vi "Streamed Data Viewer.vi"() -> ()   [LabVIEW 2013]
doc: "Use this template to build a user interface event handler design pattern. Use this pattern for dialog boxes and other user interfaces. You also can create and execute user-defined events that the VI can handle the same way as user interface events."
uses:
  <vilib>/Waveform/WDTFileIO.llb/ Write Waveforms to File (1D).vi
  <vilib>/Waveform/WDTFileIO.llb/Export Waveforms To Spreadsheet File (1D).vi
  <vilib>/Waveform/WDTOps.llb/WDT Append Waveforms DBL.vi
panel:
  in  "Save CSV Reduced":bool
  in  "Save CSV":bool
  out "Delta Y\nReduced Waveform Data":dbl format="%#.6g"
  out "Delta X\nReduced Waveform Data":dbl format="%#.6g"
  out "Delta Y\nWaveform Data":dbl format="%#.6g"
  out "Delta X\nWaveform Data":dbl format="%#.6g"
  out "offset (in bytes)":i64
  in  "Input Has Array Size":bool
  in  "Subtract":bool
  in  "Convert":bool
  out "Records\nLoaded":u32
  in  "# Channels":u32=7
  in  "End Record":u32
  in  "Start Record":u32
  in  "Save Reduced DBL":bool
  in  "Save DBL":bool
  in  "Save WFM Reduced":bool
  in  "Save WFM":bool
  in  "Reduced Data Out Directory":path
  in  "Data Out Directory":path
  in  "Reduced Records":waveform(dbl)[][](array[waveform])
  out "Reduced Waveform Data":waveform(dbl)[](graph)
  out "RF Pulse Indicies":u32[][](array[numeric])
  in  "Displayed Record":u32(slide)=1 min=1 step=1 scale=1.0..27.0
  in  "Records":waveform(dbl)[][](array[waveform])
  out "Waveform Data":waveform(dbl)[](graph)
  out "Record Count":u32
  in  "Sampling Rate":u32=500000
  in  "Record Channel Size":bool=TRUE
  in  "Path":path
  in  "Load":bool
  in  "stop":bool
  # "51200"
  # "51200 x 3"
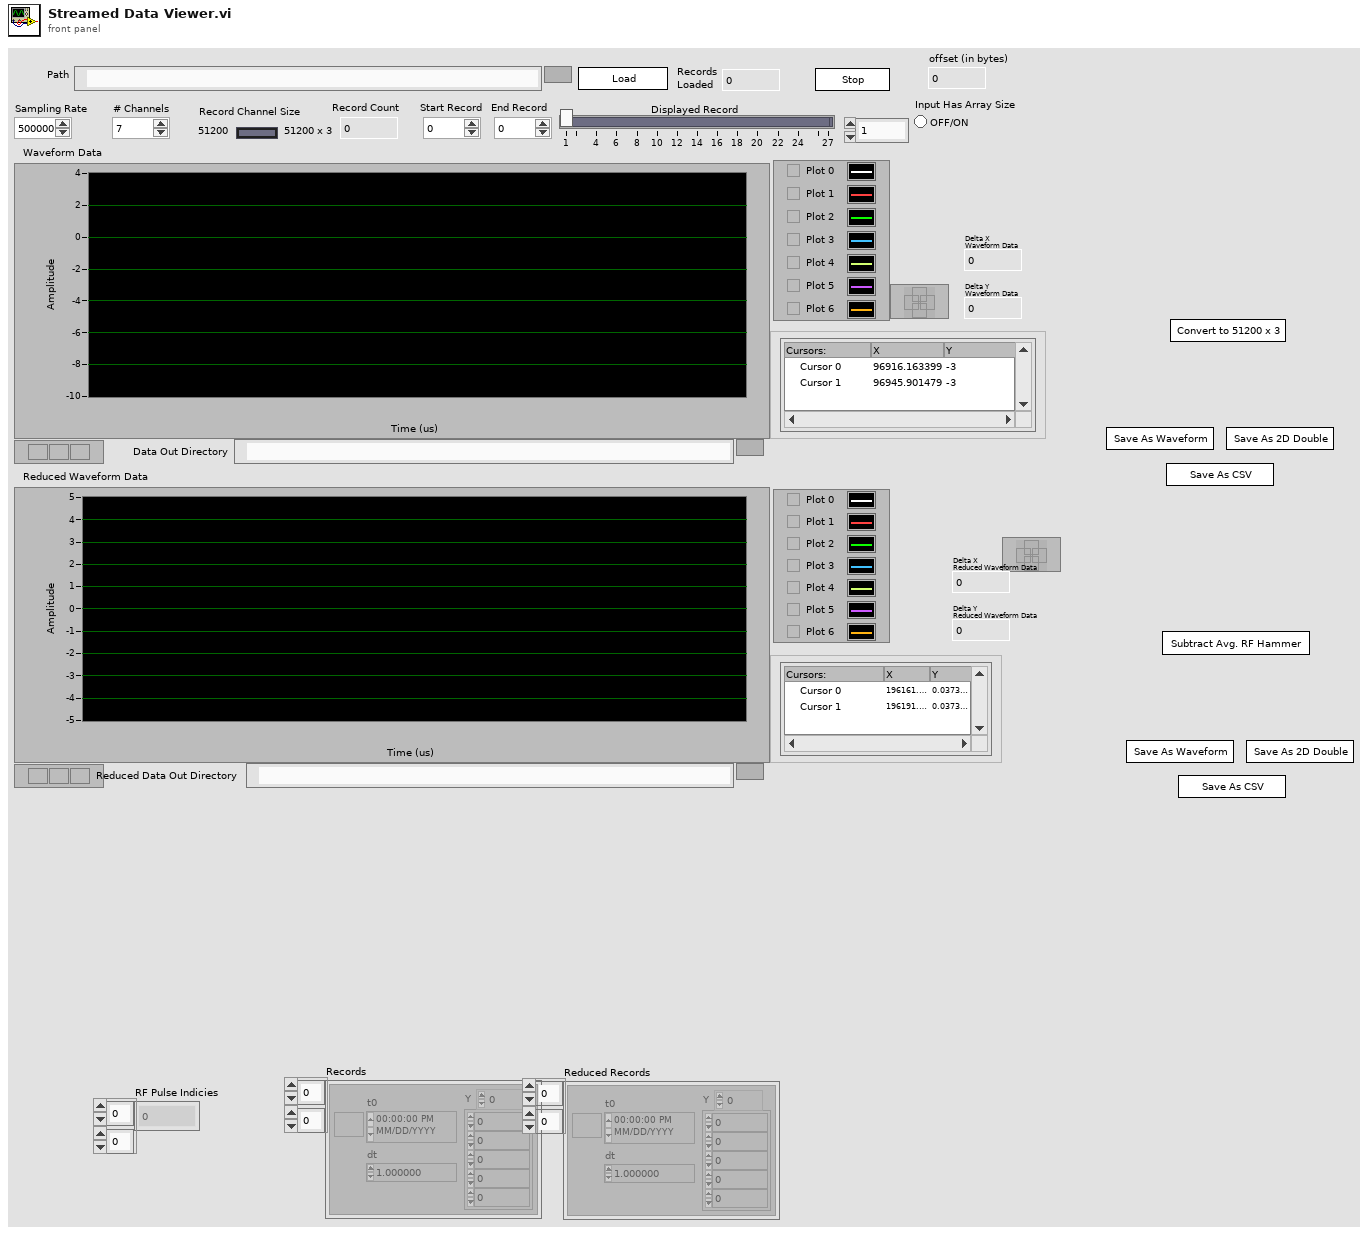
[diagram p1: front panel]
types:
  T1 = enum16{"big-endian, network order", "native, host order", "little-endian"}
  T2 = enum16{"open", "replace", "create", "open or create", "replace or create", "replace or create with confirmation"}
  T3 = typedef "LVCursorListTypeDef.ctl" = cluster{"Name":string, "Color":u32, "Style":u8, "Point Style":u8, "Name Visible":bool, "Allow Drag":bool, "Cursor Mode":u32, "Plot":i32, "Index":i32, "Position":cluster{"X":dbl, "Y":dbl}, "X Scale":u32, "Y Scale":u32, "Watch Plots":i32[], "Watch All Plots":bool, "Plot Area":i32, "Label Offset":cluster{"X":dbl, "Y":dbl}}[]
  T4 = cluster{"Name":string, "Color":u32, "Style":u8, "Point Style":u8, "Name Visible":bool, "Allow Drag":bool, "Cursor Mode":u32, "Plot":i32, "Index":i32, "Position":cluster{"X":dbl, "Y":dbl}, "X Scale":u32, "Y Scale":u32, "Watch Plots":i32[], "Watch All Plots":bool, "Plot Area":i32, "Label Offset":cluster{"X":dbl, "Y":dbl}}
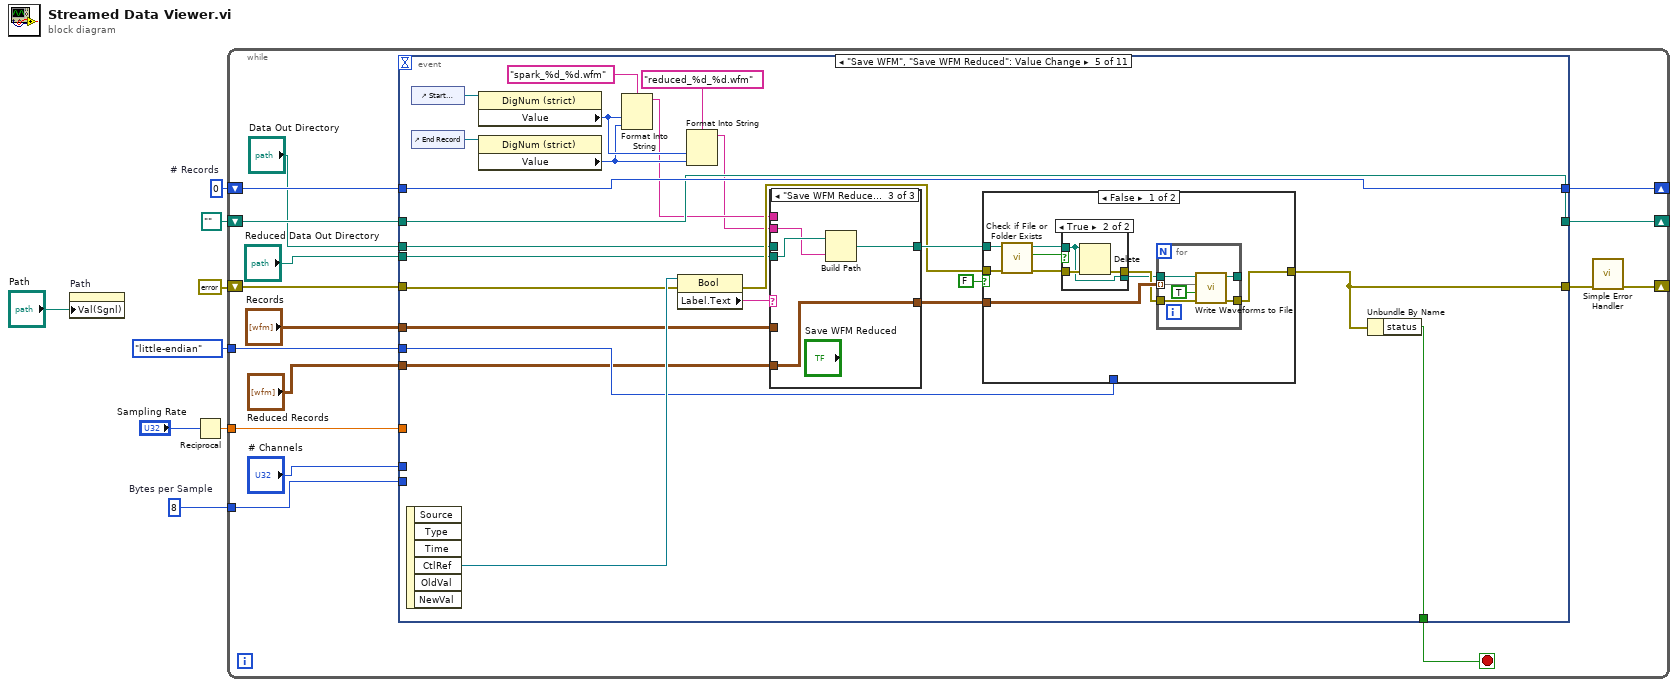
[diagram p0: block diagram]
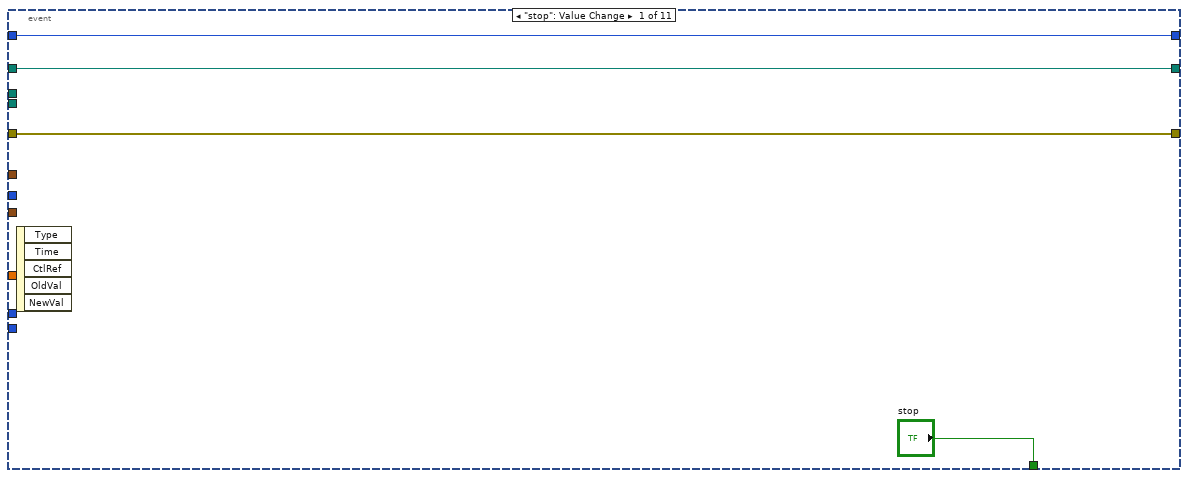
[diagram p2: hidden frame]
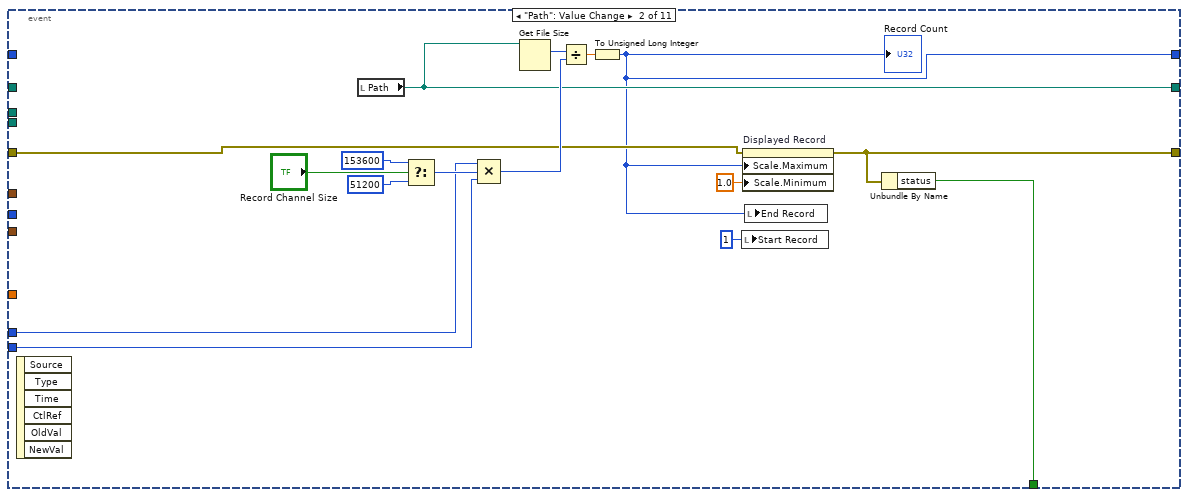
[diagram p3: hidden frame]
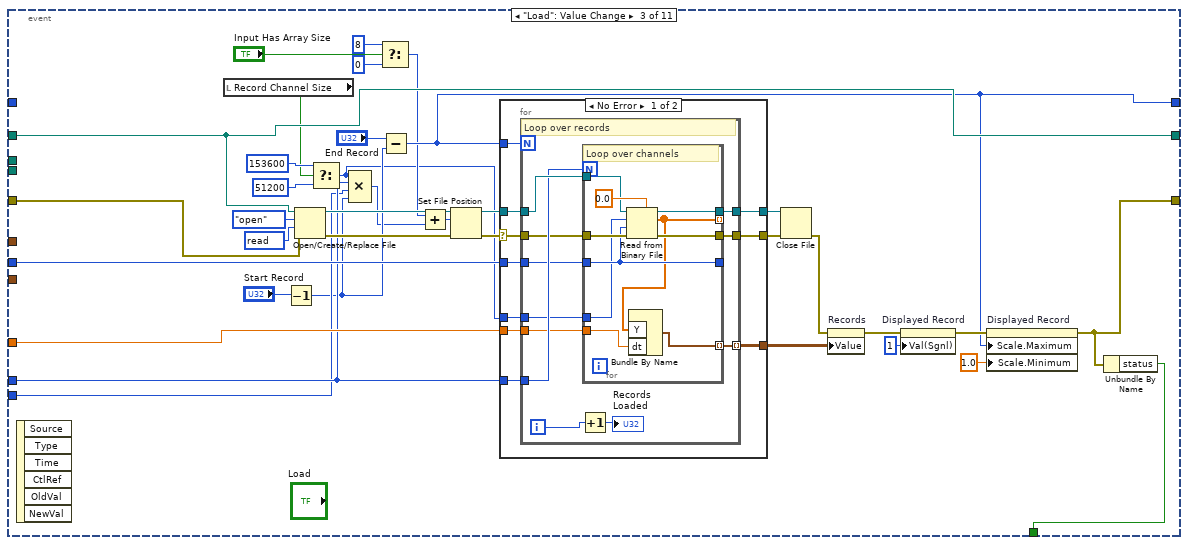
[diagram p4: hidden frame]
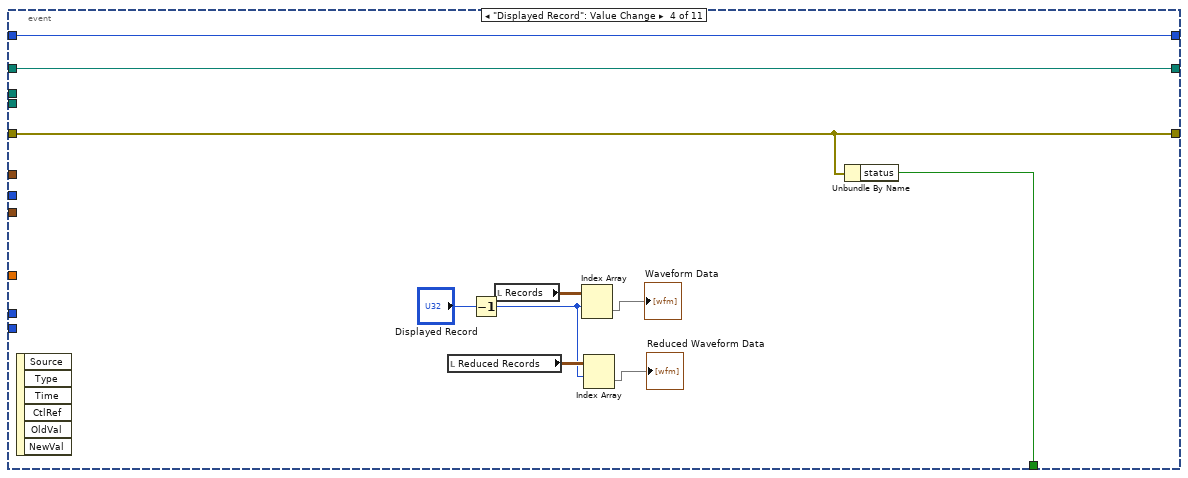
[diagram p6: hidden frame]
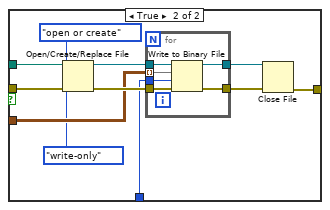
[diagram p8: hidden frame]
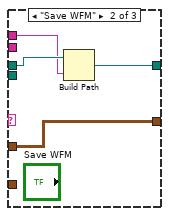
[diagram p10: hidden frame]
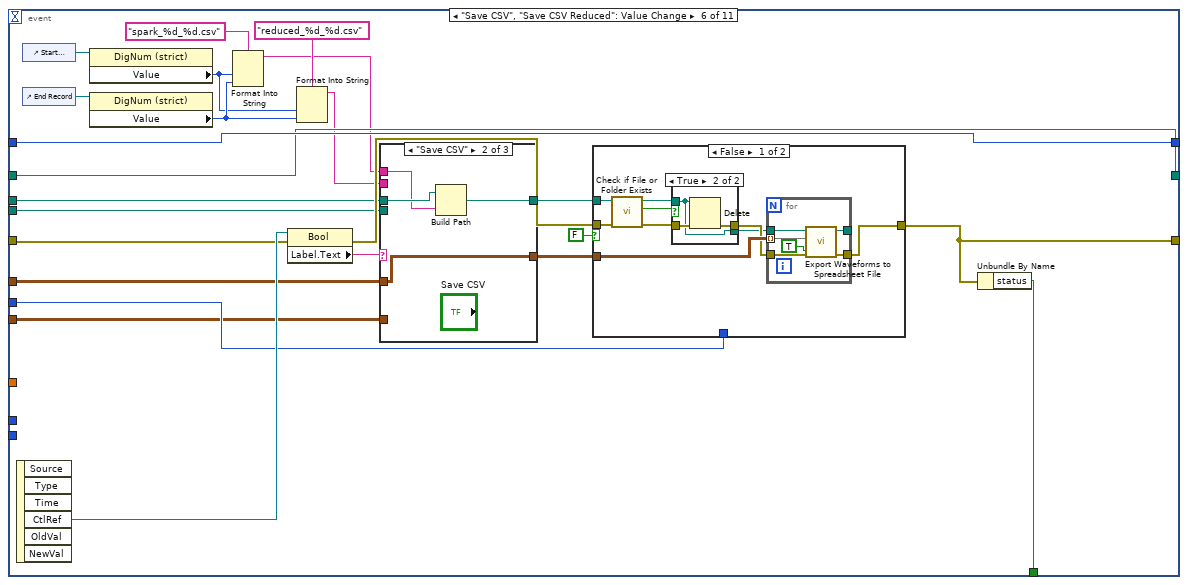
[diagram p11: hidden frame]
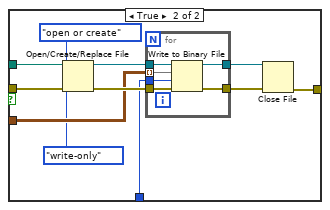
[diagram p13: hidden frame]
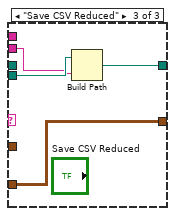
[diagram p15: hidden frame]
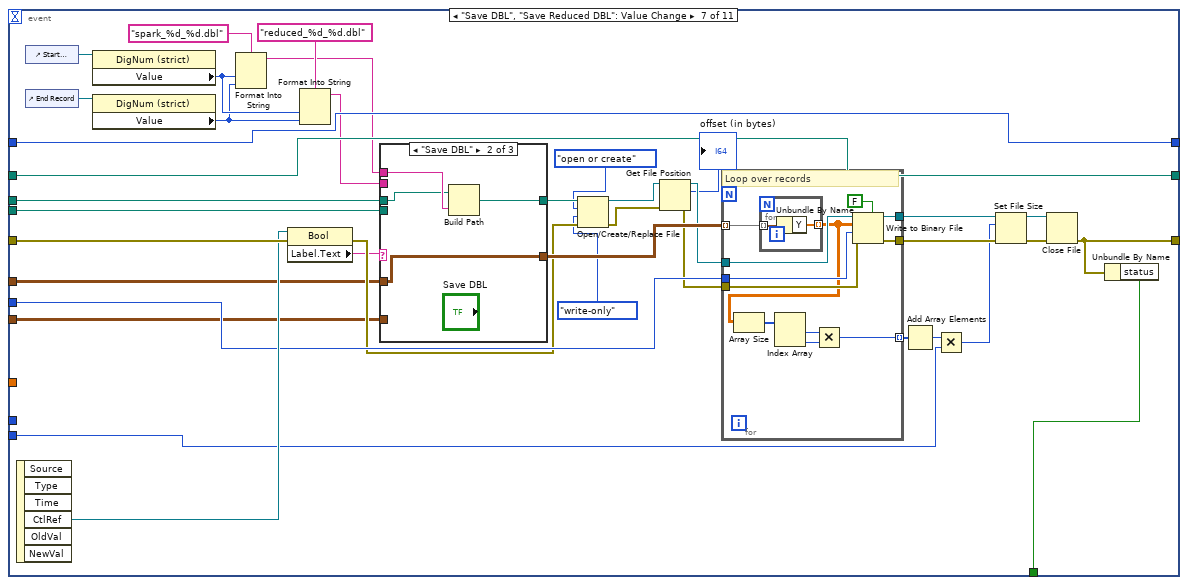
[diagram p16: hidden frame]
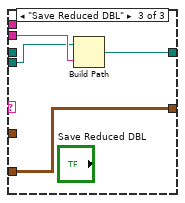
[diagram p18: hidden frame]
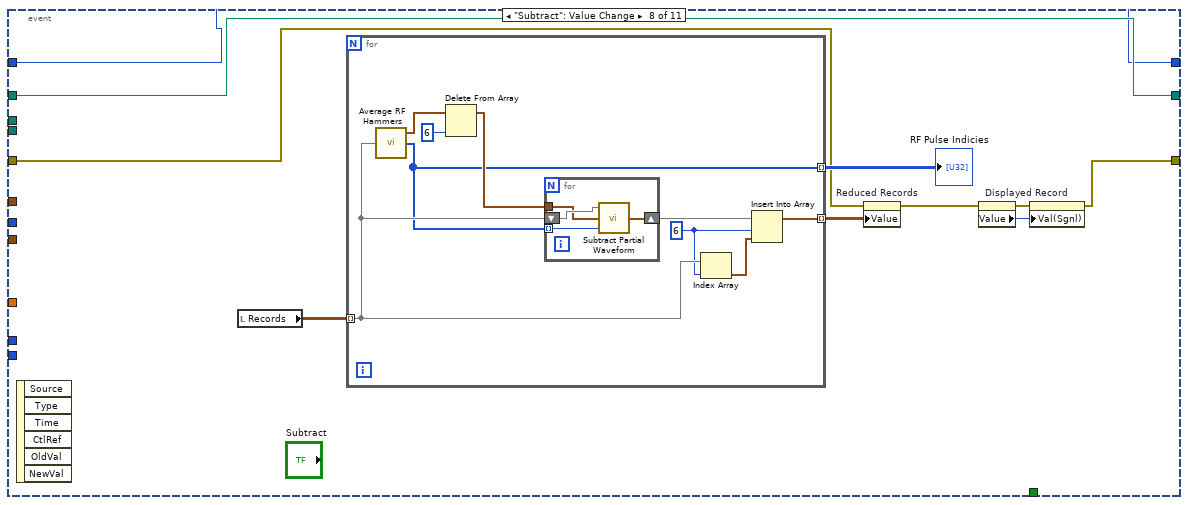
[diagram p19: hidden frame]
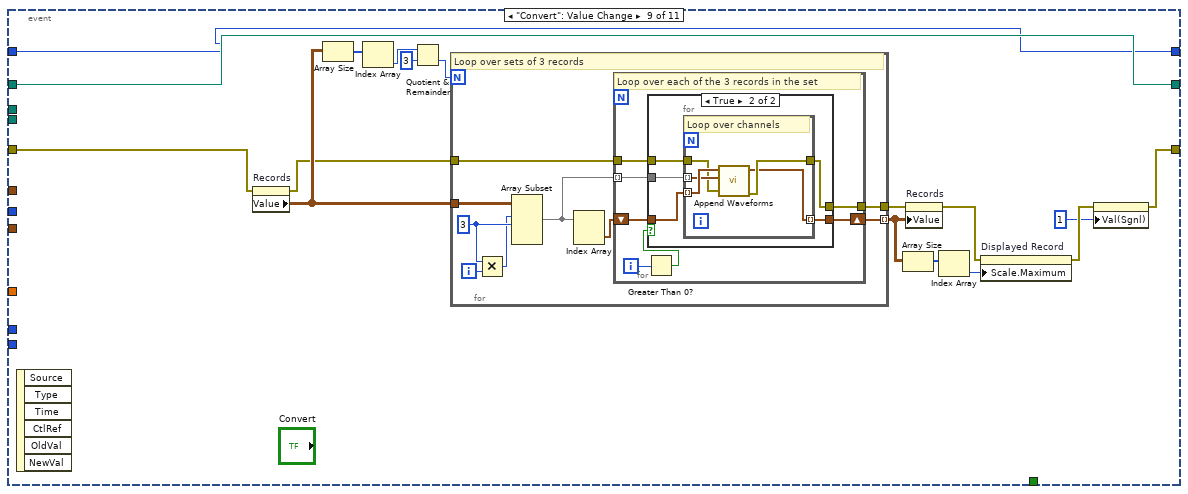
[diagram p20: hidden frame]
diagram:
  w6 = u32 8  # Bytes per Sample
  w8 = u32 0  # # Records
  n1 = property on="Path" class="Path"("Val(Sgnl)"="Path") -> ()  [unwired: 2 in, 2 out]
  n2 = Reciprocal(x="Sampling Rate") -> (1/x=w4:dbl)
  n3 = while {
    shift-right: [w23] -> _
    shift-left: w8 -> [w22]
    shift-right: [w21] -> _
    shift-left: path "" ("Path") -> [w20]
    tunnel: w6 -> [w19]
    tunnel: w4 -> [w18]
    tunnel: T1."little-endian" ("byte order (0:big-endian, network order)") -> [w17]
    shift-right: [w13] -> _
    shift-left: errorcluster {"status"=FALSE, "code"=0, "source"=""} ("error out") -> [w16]
    stop <- w24 stop-if-true
    n4 = event shown="[4] \"Save WFM\", \"Save WFM Reduced\": Value Change" {
      selector: _ -> [_ _ _ _ _ _ _ _ _ _ _]
      dyn-events: _ -> [_ _ _ _ _ _ _ _ _ _ _]
      timeout: _ -> [_ _ _ _ _ _ _ _ _ _ _]
      tunnel: ["stop" w31 w75 w114 w137 w206 w289 _ _ _ _] -> w24
      tunnel: [w26 w29 w55 w119 w141 w210 w294 w322 w353 w393 w409] -> w23
      tunnel: w22 -> [w26 _ _ w119 w141 w210 w294 w322 w353 w393 w409]
      tunnel: [w27 w37 w77 w120 w140 w209 w293 w323 w354 w392 w408] -> w21
      tunnel: w20 -> [w27 _ w77 w120 w140 w209 w293 w323 w354 w392 w408]
      tunnel: "# Channels" -> [_ w39 w64 _ _ _ _ _ _ _ _]
      tunnel: w19 -> [_ w38 w63 _ _ _ w275 _ _ _ _]
      tunnel: w18 -> [_ _ w79 _ _ _ _ _ _ _ _]
      tunnel: w17 -> [_ _ w78 _ w139 w208 w295 _ _ _ _]
      tunnel: [w25 w32 w60 w115 w138 w207 w290 w324 w355 w390 w406] -> w14
      tunnel: w16 -> [w25 w34 w71 w115 w146 w215 w299 w326 w356 w391 w407]
      tunnel: "Data Out Directory" -> [_ _ _ _ w135 w204 w273 _ _ _ _]
      tunnel: "Reduced Data Out Directory" -> [_ _ _ _ w134 w203 w272 _ _ _ _]
      tunnel: "Records" -> [_ _ _ _ w133 w202 w271 _ _ _ _]
      tunnel: "Reduced Records" -> [_ _ _ _ w132 w201 w270 _ _ _ _]
      event "stop": Value Change {
        n5 = event-data() -> ()  [unwired: 1 in, 5 out]
      }
      event "Path": Value Change {
        n6 = event-data() -> ()  [unwired: 1 in, 6 out]
        n7 = local read "Path"() -> (w37:path)
        n8 = Select(t=u32 153600, s="Record Channel Size", f=u32 51200) -> (s? t:f=w40:u32)
        n9 = Compound Arithmetic op=MULTIPLY(w39, w40, w38) -> (w41:u32)
        n10 = Get File Size(file=w37) -> (size (in bytes)=w42:i64)  [unwired: 1 in, 2 out]
        n11 = Divide(x=w42, y=w41) -> (x/y=w43:dbl)
        n12 = To Unsigned Long Integer(number=w43) -> (unsigned 32bit integer=w29:u32)
        "Record Count" <- w29
        n13 = local write "Start Record"(u32 1 ("Start Record")) -> ()
        n14 = property on="Displayed Record" class="Slide (strict)"(error in=w34, "Scale.Maximum"=w29, "Scale.Minimum"=1.0 ("Scale.Range:Minimum")) -> (error out=w32:errorcluster)  [unwired: 1 in, 1 out]
        n15 = local write "End Record"(w29) -> ()
        n16 = Unbundle By Name(w32) -> ("status"=w31:bool)
      }
      event "Load": Value Change {
        w80 = u32 2147483648 items=["read"=2147483648, "write"=1073741824, "read & write"=3221225472, "execute"=536870912, "all"=268435456] ("desired access (read & write)")
        n17 = event-data() -> ()  [unwired: 1 in, 6 out]
        n18 = local read "Record Channel Size"() -> (w65:bool)
        n19 = Decrement(x="Start Record") -> (x-1=w56:u32)
        n20 = Open/Create/Replace File(file path (use dialog)=w77, error in=w71, operation (0:open)=T2."open", access (0:read/write)=w80) -> (refnum out=w69:refnum<file>, error out=w70:errorcluster)  [unwired: 2 in, 1 out]
        n21 = Select(t=u32 153600, s=w65, f=u32 51200) -> (s? t:f=w48:u32)
        n22 = Compound Arithmetic op=MULTIPLY(w48, w64, w63, w56) -> (w50:u32)
        n23 = Select(t=u32 8, s="Input Has Array Size", f=u32 0) -> (s? t:f=w49:u32)
        n24 = Subtract(x="End Record", y=w56) -> (x-y=w55:u32)
        n25 = Add(x=w49, y=w50) -> (x+y=w51:u32)
        n26 = Set File Position(offset (in bytes) (0)=w51, refnum=w69, error in=w70) -> (refnum out=w68:refnum<file>, error out=w59:errorcluster)  [unwired: 1 in]
        n27 = case shown="No Error" w59 {
          selector: w59 -> [w81 w112]
          tunnel: w48 -> [w90 _]
          tunnel: w79 -> [w89 _]
          tunnel: w78 -> [w88 _]
          tunnel: [w87 w113] -> w47
          tunnel: [w86 _] -> w74
          tunnel: [w85 w112] -> w46
          tunnel: w68 -> [w84 w113]
          tunnel: w64 -> [w83 _]
          tunnel: w55 -> [w82 _]
          frame No Error {
            n28 = for {
              N: w82 -> [_]
              tunnel: w84 -> [w101]
              tunnel: w83 -> [w100]
              tunnel: w90 -> [w99]
              tunnel: w81 -> [w98]
              tunnel: w89 -> [w97]
              tunnel: w88 -> [w96]
              tunnel: [w95] -> w87
              tunnel: [w94] -> w85
              tunnel: [w93] -> w86 mode=indexing
              i -> [w91]
              # "Loop over records"
              n29 = Increment(x=w91) -> (x+1=→"Records\nLoaded":i32)
              n30 = for {
                N: w100 -> [_]
                tunnel: [w111] -> w93 mode=indexing
                tunnel: w101 -> [w109]
                tunnel: w99 -> [w103]
                tunnel: w98 -> [w108]
                tunnel: w97 -> [w107]
                tunnel: w96 -> [w105]
                tunnel: [w106] -> w94
                tunnel: [w105] -> _
                tunnel: [w104] -> w95
                tunnel: [w102] -> _ mode=indexing
                # "Loop over channels"
                n31 = Read from Binary File(5:0.0, 8:w108, 9:w105, 10:w103, 11:w109) -> (0:w106:errorcluster, 2:w102:dbl[], 3:w104:refnum<file>)  [unwired: 1 in, 1 out]
                n32 = Bundle By Name("Y"=w102, "dt"=w107) -> (w111:waveform(dbl))  [unwired: 1 in]
              }
            }
          }
          frame Error {
          }
        }
        n33 = Close File(refnum=w47, error in=w46) -> (error out=w45:errorcluster)  [unwired: 1 out]
        n34 = property on="Records" class="Arr (strict)"(error in=w45, "Value"=w74) -> (error out=w72:errorcluster)  [unwired: 1 in, 1 out]
        n35 = property on="Displayed Record" class="Slide (strict)"(error in=w72, "Val(Sgnl)"=u32 1 ("Value (Signaling)")) -> (error out=w61:errorcluster)  [unwired: 1 in, 1 out]
        n36 = property on="Displayed Record" class="Slide (strict)"(error in=w61, "Scale.Maximum"=w55, "Scale.Minimum"=1.0 ("Scale.Range:Minimum")) -> (error out=w60:errorcluster)  [unwired: 1 in, 1 out]
        n37 = Unbundle By Name(w60) -> ("status"=w75:bool)
      }
      event "Displayed Record": Value Change {
        n38 = event-data() -> ()  [unwired: 1 in, 6 out]
        n39 = local read "Reduced Records"() -> (w118:waveform(dbl)[][])
        n40 = Decrement(x="Displayed Record") -> (x-1=w117:u32)
        n41 = local read "Records"() -> (w123:waveform(dbl)[][])
        n42 = Index Array(array=w123, index (row)=w117) -> (element=→"Waveform Data":waveform(dbl)[])  [unwired: 1 in]
        n43 = Index Array(array=w118, index (row)=w117) -> (element=→"Reduced Waveform Data":waveform(dbl)[])  [unwired: 1 in]
        n44 = Unbundle By Name(w115) -> ("status"=w114:bool)
      }
      event "Save WFM", "Save WFM Reduced": Value Change {
        n45 = event-data() -> ("CtlRef"=w147:refnum<vi>)  [unwired: 1 in, 5 out]
        n46 = control-ref of="Start Record"() -> (w131:refnum<vi>)
        n47 = control-ref of="End Record"() -> (w130:refnum<vi>)
        n48 = property class="DigNum (strict)"(reference=w131) -> ("Value"=w127:u32)  [unwired: 1 in, 2 out]
        n49 = property class="DigNum (strict)"(reference=w130) -> ("Value"=w126:u32)  [unwired: 1 in, 2 out]
        n50 = Format Into String(format string="spark_%d_%d.wfm", w127, w126) -> (resulting string=w125:string)  [unwired: 2 in, 1 out]
        n51 = property class="Bool"(reference=w147, error in=w146) -> (error out=w143:errorcluster, "Label.Text"=w145:string)  [unwired: 1 out]
        n52 = Format Into String(format string="reduced_%d_%d.wfm", w127, w126) -> (resulting string=w124:string)  [unwired: 2 in, 1 out]
        n53 = case shown="\"Save WFM Reduced\"" w145 {
          tunnel: [_ w185 w189] -> w144
          tunnel: [_ w188 w192] -> w142
          tunnel: w135 -> [_ w187 _]
          tunnel: w134 -> [_ _ w191]
          tunnel: w133 -> [_ w188 _]
          tunnel: w132 -> [_ _ w192]
          tunnel: w125 -> [_ w186 _]
          tunnel: w124 -> [_ _ w190]
          frame Default {
            # "NO-OP"
          }
          frame "Save WFM" {
            n54 = Build Path(base path=w187, name or relative path=w186) -> (appended path=w185:path)
          }
          frame "Save WFM Reduced" {
            n55 = Build Path(base path=w191, name or relative path=w190) -> (appended path=w189:path)
          }
        }
        n56 = case shown="False" FALSE {
          tunnel: w144 -> [w151 w178]
          tunnel: w143 -> [w152 w177]
          tunnel: w142 -> [w156 w175]
          tunnel: w139 -> [_ w171]
          tunnel: [w154 w170] -> w138
          frame False {
            n57 = call <vilib>:"Check if File or Folder Exists.vi"("error in (no error)"=w152, "path"=w151) -> ("error out"=w149:errorcluster, "file or folder exists?"=w148:bool, "dup path"=w150:path)  [unwired: 7 in]
            n58 = case shown="True" w148 {
              tunnel: w150 -> [w157 w159]
              tunnel: w149 -> [w158 w161]
              tunnel: [w157 w159] -> w153
              tunnel: [w158 w160] -> w155
              frame False {
              }
              frame True {
                n59 = Delete(path (use dialog)=w159, error in=w161) -> (error out=w160:errorcluster)  [unwired: 3 in, 2 out]
              }
            }
            n60 = for {
              tunnel: w155 -> [w167]
              tunnel: w156 -> [w163] mode=indexing
              tunnel: [w166] -> w154
              tunnel: [w165] -> _
              tunnel: w153 -> [w164]
              n61 = call-poly <vilib>:"Write Waveforms to File.vi"("error in (no error)"=w167, "append to file? (new file:F)"=TRUE, "waveform array"=w163, "file path (dialog if empty)"=w164) -> ("error out"=w166:errorcluster, "new file path (Not A Path if cancelled)"=w165:path)  [unwired: 6 in]
            }
          }
          frame True {
            n62 = Open/Create/Replace File(file path (use dialog)=w178, error in=w177, operation (0:open)=T2."open or create", access (0:read/write)=enum16{"read/write", "read-only", "write-only"}."write-only") -> (refnum out=w172:refnum<file>, error out=w176:errorcluster)  [unwired: 2 in, 1 out]
            n63 = for {
              tunnel: w176 -> [w184]
              tunnel: w175 -> [w183] mode=indexing
              tunnel: [w182] -> w174
              tunnel: [w181] -> w173
              tunnel: w172 -> [w180]
              tunnel: w171 -> [w179]
              n64 = Write to Binary File(file (use dialog)=w180, data=w183, error in=w184, 9:w179) -> (refnum out=w181:refnum<file>, error out=w182:errorcluster)  [unwired: 2 in, 1 out]
            }
            n65 = Close File(refnum=w173, error in=w174) -> (error out=w170:errorcluster)  [unwired: 1 out]
          }
        }
        n66 = Unbundle By Name(w138) -> ("status"=w137:bool)
      }
      event "Save CSV", "Save CSV Reduced": Value Change {
        n67 = event-data() -> ("CtlRef"=w216:refnum<vi>)  [unwired: 1 in, 5 out]
        n68 = control-ref of="Start Record"() -> (w196:refnum<vi>)
        n69 = control-ref of="End Record"() -> (w197:refnum<vi>)
        n70 = property class="DigNum (strict)"(reference=w196) -> ("Value"=w199:u32)  [unwired: 1 in, 2 out]
        n71 = property class="DigNum (strict)"(reference=w197) -> ("Value"=w200:u32)  [unwired: 1 in, 2 out]
        n72 = Format Into String(format string="spark_%d_%d.csv", w199, w200) -> (resulting string=w195:string)  [unwired: 2 in, 1 out]
        n73 = property class="Bool"(reference=w216, error in=w215) -> (error out=w212:errorcluster, "Label.Text"=w214:string)  [unwired: 1 out]
        n74 = Format Into String(format string="reduced_%d_%d.csv", w199, w200) -> (resulting string=w194:string)  [unwired: 2 in, 1 out]
        n75 = case shown="\"Save CSV\"" w214 {
          tunnel: [_ w256 w260] -> w213
          tunnel: [_ w257 w261] -> w211
          tunnel: w204 -> [_ w255 _]
          tunnel: w203 -> [_ _ w259]
          tunnel: w202 -> [_ w257 _]
          tunnel: w201 -> [_ _ w261]
          tunnel: w195 -> [_ w254 _]
          tunnel: w194 -> [_ _ w258]
          frame Default {
            # "NO-OP"
          }
          frame "Save CSV" {
            n76 = Build Path(base path=w255, name or relative path=w254) -> (appended path=w256:path)
          }
          frame "Save CSV Reduced" {
            n77 = Build Path(base path=w259, name or relative path=w258) -> (appended path=w260:path)
          }
        }
        n78 = case shown="False" FALSE {
          tunnel: w213 -> [w220 w247]
          tunnel: w212 -> [w221 w246]
          tunnel: w211 -> [w225 w244]
          tunnel: w208 -> [_ w240]
          tunnel: [w223 w239] -> w207
          frame False {
            n79 = call <vilib>:"Check if File or Folder Exists.vi"("error in (no error)"=w221, "path"=w220) -> ("error out"=w218:errorcluster, "file or folder exists?"=w217:bool, "dup path"=w219:path)  [unwired: 7 in]
            n80 = case shown="True" w217 {
              tunnel: w219 -> [w226 w228]
              tunnel: w218 -> [w227 w230]
              tunnel: [w226 w228] -> w222
              tunnel: [w227 w229] -> w224
              frame False {
              }
              frame True {
                n81 = Delete(path (use dialog)=w228, error in=w230) -> (error out=w229:errorcluster)  [unwired: 3 in, 2 out]
              }
            }
            n82 = for {
              tunnel: w224 -> [w236]
              tunnel: w225 -> [w232] mode=indexing
              tunnel: [w235] -> w223
              tunnel: [w234] -> _
              tunnel: w222 -> [w233]
              n83 = call-poly <vilib>:"Export Waveforms to Spreadsheet File.vi"("append to file? (new file:F)"=TRUE, "error in (no error)"=w236, "waveforms"=w232, "file path (dialog if empty)"=w233) -> ("error out"=w235:errorcluster, "new file path (Not A Path if cancelled)"=w234:path)  [unwired: 6 in]
            }
          }
          frame True {
            n84 = Open/Create/Replace File(file path (use dialog)=w247, error in=w246, operation (0:open)=T2."open or create", access (0:read/write)=enum16{"read/write", "read-only", "write-only"}."write-only") -> (refnum out=w241:refnum<file>, error out=w245:errorcluster)  [unwired: 2 in, 1 out]
            n85 = for {
              tunnel: w245 -> [w253]
              tunnel: w244 -> [w252] mode=indexing
              tunnel: [w251] -> w243
              tunnel: [w250] -> w242
              tunnel: w241 -> [w249]
              tunnel: w240 -> [w248]
              n86 = Write to Binary File(file (use dialog)=w249, data=w252, error in=w253, 9:w248) -> (refnum out=w250:refnum<file>, error out=w251:errorcluster)  [unwired: 2 in, 1 out]
            }
            n87 = Close File(refnum=w242, error in=w243) -> (error out=w239:errorcluster)  [unwired: 1 out]
          }
        }
        n88 = Unbundle By Name(w207) -> ("status"=w206:bool)
      }
      event "Save DBL", "Save Reduced DBL": Value Change {
        n89 = event-data() -> ("CtlRef"=w298:refnum<vi>)  [unwired: 1 in, 5 out]
        n90 = control-ref of="Start Record"() -> (w268:refnum<vi>)
        n91 = control-ref of="End Record"() -> (w267:refnum<vi>)
        n92 = property class="DigNum (strict)"(reference=w268) -> ("Value"=w265:u32)  [unwired: 1 in, 2 out]
        n93 = property class="DigNum (strict)"(reference=w267) -> ("Value"=w264:u32)  [unwired: 1 in, 2 out]
        n94 = Format Into String(format string="spark_%d_%d.dbl", w265, w264) -> (resulting string=w263:string)  [unwired: 2 in, 1 out]
        n95 = property class="Bool"(reference=w298, error in=w299) -> (error out=w292:errorcluster, "Label.Text"=w291:string)  [unwired: 1 out]
        n96 = Format Into String(format string="reduced_%d_%d.dbl", w265, w264) -> (resulting string=w262:string)  [unwired: 2 in, 1 out]
        n97 = case shown="\"Save DBL\"" w291 {
          tunnel: [_ w316 w320] -> w297
          tunnel: [_ w317 w321] -> w296
          tunnel: w273 -> [_ w314 _]
          tunnel: w272 -> [_ _ w318]
          tunnel: w271 -> [_ w317 _]
          tunnel: w270 -> [_ _ w321]
          tunnel: w263 -> [_ w315 _]
          tunnel: w262 -> [_ _ w319]
          frame Default {
            # "NO-OP"
          }
          frame "Save DBL" {
            n98 = Build Path(base path=w314, name or relative path=w315) -> (appended path=w316:path)
          }
          frame "Save Reduced DBL" {
            n99 = Build Path(base path=w318, name or relative path=w319) -> (appended path=w320:path)
          }
        }
        n100 = Open/Create/Replace File(file path (use dialog)=w297, error in=w292, operation (0:open)=T2."open or create", access (0:read/write)=enum16{"read/write", "read-only", "write-only"}."write-only") -> (refnum out=w285:refnum<file>, error out=w284:errorcluster)  [unwired: 2 in, 1 out]
        n101 = Get File Position(4:w284, 7:w285) -> (0:w283:errorcluster, 2:→"offset (in bytes)":i64, 3:w286:refnum<file>)
        n102 = for {
          tunnel: w283 -> [w311]
          tunnel: w296 -> [w306] mode=indexing
          tunnel: [w310] -> w279
          tunnel: [w309] -> w280
          tunnel: w286 -> [w308]
          tunnel: w295 -> [w307]
          tunnel: [w300] -> w281 mode=indexing
          # "Loop over records"
          n103 = for {
            tunnel: w306 -> [w313] mode=indexing
            tunnel: [w312] -> w304 mode=indexing
            n104 = Unbundle By Name(w313) -> ("Y"=w312:dbl[])
          }
          n105 = Array Size(array=w304) -> (size(s)=w303:i32[])
          n106 = Index Array(array=w303) -> (element #1=w301:i32, element #2=w302:i32)  [unwired: 2 in]
          n107 = Multiply(x=w301, y=w302) -> (x*y=w300:i32)
          n108 = Write to Binary File(file (use dialog)=w308, data=w304, error in=w311, 5:FALSE ("prepend array or string size? (T)"), 9:w307) -> (refnum out=w309:refnum<file>, error out=w310:errorcluster)  [unwired: 1 in, 1 out]
        }
        n109 = Add Array Elements(numeric array=w281) -> (sum=w276:i32)
        n110 = Multiply(x=w276, y=w275) -> (x*y=w274:u32)
        n111 = Set File Size(4:w279, 6:w274, 7:w280) -> (0:w278:errorcluster, 3:w277:refnum<file>)
        n112 = Close File(refnum=w277, error in=w278) -> (error out=w290:errorcluster)  [unwired: 1 out]
        n113 = Unbundle By Name(w290) -> ("status"=w289:bool)
      }
      event "Subtract": Value Change {
        n114 = event-data() -> ()  [unwired: 1 in, 6 out]
        n115 = local read "Records"() -> (w331:waveform(dbl)[][])
        n116 = for {
          tunnel: w331 -> [w335] mode=indexing
          tunnel: [w333] -> w330 mode=indexing
          tunnel: [w332] -> w327 mode=indexing
          w334 = 6 ("index")
          n117 = call "Average RF Hammers.vi"("Record"=w335) -> ("RF Pulse Start Indicies"=w333:u32[], "Waveform Graph"=w340:waveform(dbl)[])  [unwired: 2 in, 1 out]
          n118 = Delete From Array(array=w340, index=6) -> (array with subset deleted=w339:waveform(dbl)[])  [unwired: 1 in, 1 out]
          n119 = for {
            tunnel: w339 -> [w343]
            tunnel: w333 -> [w341] mode=indexing
            shift-right: [w342] -> w338
            shift-left: w335 -> [w344]
            n120 = call "Subtract Partial Waveform.vi"("Offset (0)"=w341, "Subsignal"=w343, "Signal"=w344) -> ("Difference"=w342:waveform(dbl)[])  [unwired: 2 in]
          }
          n121 = Index Array(array=w335, index=w334) -> (element=w336:waveform(dbl))
          n122 = Insert Into Array(array=w338, index=w334, new element=w336) -> (w332:waveform(dbl)[])
        }
        "RF Pulse Indicies" <- w330
        n123 = property on="Reduced Records" class="Arr (strict)"(error in=w326, "Value"=w327) -> (error out=w325:errorcluster)  [unwired: 1 in, 1 out]
        n124 = property on="Displayed Record" class="Slide (strict)"(error in=w325) -> (error out=w328:errorcluster, "Value"=w329:u32)  [unwired: 1 in, 1 out]
        n125 = property on="Displayed Record" class="Slide (strict)"(error in=w328, "Val(Sgnl)"=w329) -> (error out=w324:errorcluster)  [unwired: 1 in, 1 out]
      }
      event "Convert": Value Change {
        n126 = event-data() -> ()  [unwired: 1 in, 6 out]
        n127 = property on="Records" class="Arr (strict)"(error in=w356) -> (error out=w352:errorcluster, "Value"=w357:waveform(dbl)[][])  [unwired: 1 in, 1 out]
        n128 = Array Size(array=w357) -> (size(s)=w361:i32[])
        n129 = Index Array(array=w361) -> (element=w360:i32)  [unwired: 1 in]
        n130 = Quotient & Remainder(x=w360, y=3) -> (floor(x/y)=w358:i32)  [unwired: 1 out]
        n131 = for {
          N: w358 -> [_]
          tunnel: w357 -> [w370]
          tunnel: [w362] -> w350 mode=indexing
          tunnel: w352 -> [w364]
          tunnel: [w363] -> w351
          i -> [w369]
          w368 = 3 ("length")
          # "Loop over sets of 3 records"
          n132 = Multiply(x=w368, y=w369) -> (x*y=w367:i32)
          n133 = Array Subset(array=w370, index (row)=w367, length (row)=w368) -> (w365:waveform(dbl)[][])  [unwired: 2 in]
          n134 = Index Array(array=w365) -> (element=w366:waveform(dbl)[])  [unwired: 2 in]
          n135 = for {
            tunnel: w365 -> [w374] mode=indexing
            shift-right: [w373] -> w362
            shift-left: w366 -> [w375]
            tunnel: w364 -> [w372]
            tunnel: [w371] -> w363
            i -> [w377]
            # "Loop over each of the 3 records in the set"
            n136 = Greater Than 0?(x=w377) -> (x > 0?=w376:bool)
            n137 = case shown="True" w376 {
              tunnel: w375 -> [w379 w383]
              tunnel: w374 -> [_ w384]
              tunnel: [w379 w380] -> w373
              tunnel: w372 -> [w378 w382]
              tunnel: [w378 w381] -> w371
              frame False {
              }
              frame True {
                n138 = for {
                  tunnel: w384 -> [w388] mode=indexing
                  tunnel: w383 -> [w389] mode=indexing
                  tunnel: w382 -> [w387]
                  tunnel: [w386] -> w381
                  tunnel: [w385] -> w380 mode=indexing
                  # "Loop over channels"
                  n139 = call-poly <vilib>:"Append Waveforms.vi"("error in (no error)"=w387, "waveform B"=w388, "waveform A"=w389) -> ("error out"=w386:errorcluster, "waveform out"=w385:waveform(dbl))  [unwired: 7 in]
                }
              }
            }
          }
        }
        n140 = Array Size(array=w350) -> (size(s)=w348:i32[])
        n141 = property on="Records" class="Arr (strict)"(error in=w351, "Value"=w350) -> (error out=w347:errorcluster)  [unwired: 1 in, 1 out]
        n142 = Index Array(array=w348) -> (element=w349:i32)  [unwired: 1 in]
        n143 = property on="Displayed Record" class="Slide (strict)"(error in=w347, "Scale.Maximum"=w349) -> (error out=w346:errorcluster)  [unwired: 1 in, 1 out]
        n144 = property on="Displayed Record" class="Slide (strict)"(error in=w346, "Val(Sgnl)"=u32 1 ("Value (Signaling)")) -> (error out=w355:errorcluster)  [unwired: 1 in, 1 out]
      }
      event "Waveform Data": Cursor Move {
        n145 = event-data() -> ("CtlRef"=w403:refnum<vi>)  [unwired: 1 in, 5 out]
        n146 = property class="WFGraph (strict)"(reference=w403, error in=w391) -> (error out=w390:errorcluster, "CrsrList"=w402:T3)  [unwired: 1 out]
        n147 = Index Array(array=w402) -> (element #1=w401:T4, element #2=w400:T4)  [unwired: 2 in]
        n148 = Unbundle By Name(w400) -> ("Position.X"=w399:dbl, "Position.Y"=w396:dbl)
        n149 = Unbundle By Name(w401) -> ("Position.X"=w398:dbl, "Position.Y"=w397:dbl)
        n150 = Subtract(x=w399, y=w398) -> (x-y=→"Delta X\nWaveform Data":dbl)
        n151 = Subtract(x=w396, y=w397) -> (x-y=→"Delta Y\nWaveform Data":dbl)
      }
      event "Reduced Waveform Data": Cursor Move {
        n152 = event-data() -> ("CtlRef"=w417:refnum<vi>)  [unwired: 1 in, 5 out]
        n153 = property class="WFGraph (strict)"(reference=w417, error in=w407) -> (error out=w406:errorcluster, "CrsrList"=w416:T3)  [unwired: 1 out]
        n154 = Index Array(array=w416) -> (element #1=w415:T4, element #2=w414:T4)  [unwired: 2 in]
        n155 = Unbundle By Name(w414) -> ("Position.X"=w413:dbl, "Position.Y"=w410:dbl)
        n156 = Unbundle By Name(w415) -> ("Position.X"=w412:dbl, "Position.Y"=w411:dbl)
        n157 = Subtract(x=w413, y=w412) -> (x-y=→"Delta X\nReduced Waveform Data":dbl)
        n158 = Subtract(x=w410, y=w411) -> (x-y=→"Delta Y\nReduced Waveform Data":dbl)
      }
    }
    n159 = call <vilib>:"Simple Error Handler.vi"("error in (no error)"=w14) -> ("error out"=w13:errorcluster)  [unwired: 4 in, 4 out]
  }
